vi "生成异或校验字.vi"(11 "字符串":string="$12038") -> (2 "异或和":string, 3 "连接的字符串":string)   [LabVIEW 2017]
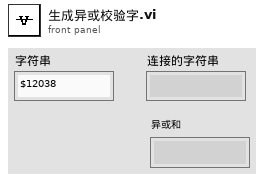
[diagram p1: front panel]
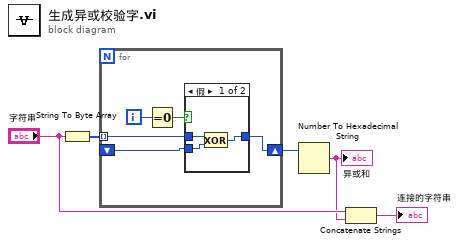
[diagram p0: block diagram]
diagram:
  n1 = String To Byte Array(string="字符串") -> (unsigned byte array=w5:u8[])
  n2 = for {
    tunnel: w5 -> [w8] mode=indexing
    shift-right: [w7] -> w4
    shift-left: _ -> [w6]
    i -> [w10]
    n3 = Equal To 0?(x=w10) -> (x = 0?=w9:bool)
    n4 = case shown="假" w9 {
      tunnel: w8 -> [w13 w14]
      tunnel: [w12 w14] -> w7
      tunnel: w6 -> [w11 _]
      frame False {
        n5 = Exclusive Or(1:w11, 2:w13) -> (0:w12:u8)
      }
      frame True {
      }
    }
  }
  n6 = Number To Hexadecimal String(2:w4) -> (0:w2:string)  [unwired: 1 in]
  "异或和" <- w2
  n7 = Concatenate Strings("字符串", w2) -> (→"连接的字符串":string)
